vi "NR_REMap.vi"(2 "Nu":dbl, 3 "prb_num":dbl, 4 "DMRS_symbol":dbl, 5 "Second_DMRS_L":dbl, 6 "rsdata":cxt[][](array[numeric]), 7 "Nsym_slot":dbl, 8 "error in (no error)":errorcluster caption="错误输入（无错误）", 9 "Frist_DMRS_L0":dbl, 10 "precodedata":cdb[](array[numeric]), 11 "appended path":path) -> (0 "error IO":errorcluster, 1 "fredata":cdb[][](array[numeric]))   [LabVIEW 2015]
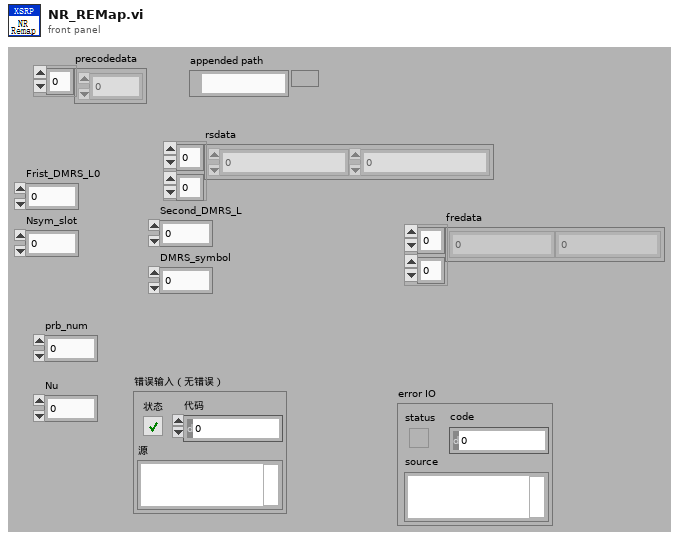
[diagram p1: front panel]
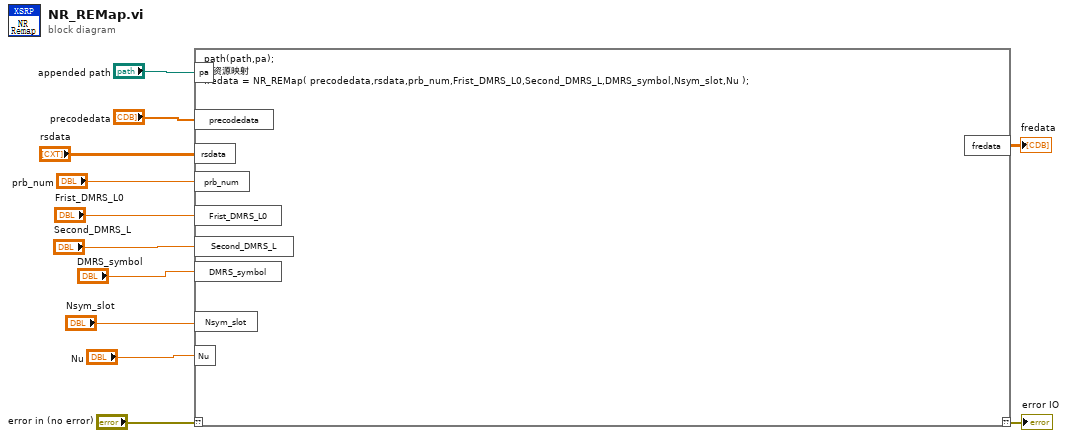
[diagram p0: block diagram]
diagram:
  n1 = script code="path(path,pa);\n%资源映射\nfredata = NR_REMap( precodedata,rsdata,prb_num,Frist_DMRS_L0,Second_DMRS_L,DMRS_symbol,Nsym_slot,Nu );"("??"="error in (no error)", "pa"="appended path", "precodedata"="precodedata", "Frist_DMRS_L0"="Frist_DMRS_L0", "Nsym_slot"="Nsym_slot", "prb_num"="prb_num", "Nu"="Nu", "rsdata"="rsdata", "Second_DMRS_L"="Second_DMRS_L", "DMRS_symbol"="DMRS_symbol") -> ("??"=→"error IO":errorcluster, "fredata"=→"fredata":cdb[][])
